vi "Move.vi"(8 "error in (no error)":errorcluster, 11 "Snake in":refnum<class "Snake.lvclass">) -> (0 "error out":errorcluster, 3 "Snake out":refnum<class "Snake.lvclass">)   [LabVIEW 2019, in "RT_Game.lvlib" / "Snake.lvclass"]
uses:
  Snake.lvclass
  Snake.lvclass/Snake.ctl
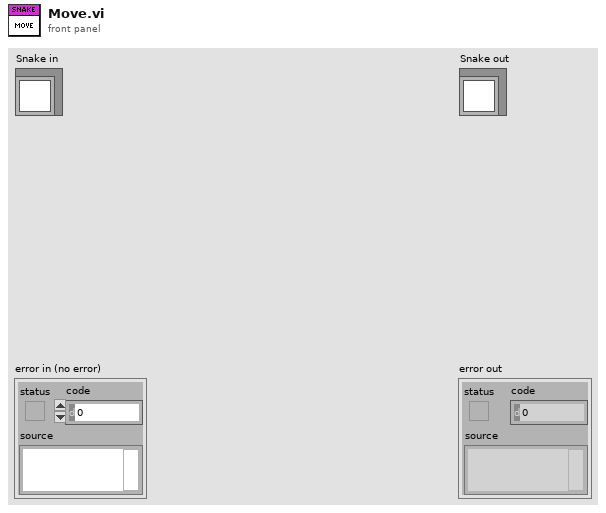
[diagram p1: front panel]
types:
  T1 = typedef "RT_Game.lvlib/Game.lvclass/Coordinate.ctl" = cluster{"x":i16, "y":i16}
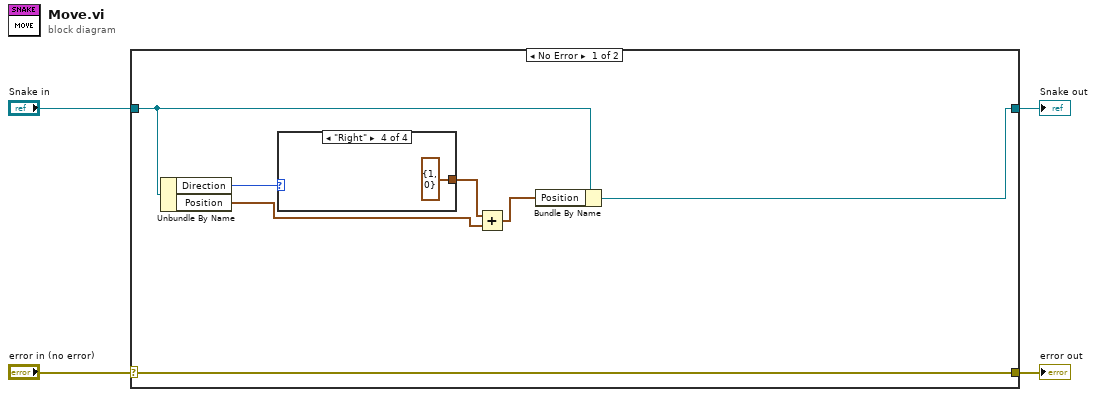
[diagram p0: block diagram]
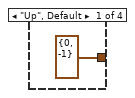
[diagram p2: hidden frame]
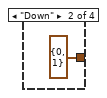
[diagram p3: hidden frame]
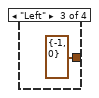
[diagram p4: hidden frame]
diagram:
  n1 = case shown="No Error" "error in (no error)" {
    selector: "error in (no error)" -> [w11 w17]
    tunnel: [w11 w17] -> w3
    tunnel: [w8 w16] -> w1
    tunnel: "Snake in" -> [w10 w16]
    frame No Error {
      n2 = Unbundle By Name(w10) -> ("Direction"=w9:enum16{"Up", "Down", "Left", "Right"}, "Position"=w7:T1)
      n3 = case shown="\"Right\"" w9 {
        tunnel: [cluster{"x":i8, "y":i8} {"x"=0, "y"=-1} ("x") cluster{"x":i8, "y":i8} {"x"=0, "y"=1} ("x") cluster{"x":i8, "y":i8} {"x"=-1, "y"=0} ("x") cluster{"x":i8, "y":i8} {"x"=1, "y"=0} ("x")] -> w6
        frame "Up", Default {
        }
        frame "Down" {
        }
        frame "Left" {
        }
        frame "Right" {
        }
      }
      n4 = Add(x=w6, y=w7) -> (x+y=w5:T1)
      n5 = Bundle By Name(cluster=w10, "Position"=w5) -> (w8:refnum<class "Snake.lvclass">)
    }
    frame Error {
    }
  }
  "error out" <- w3
  "Snake out" <- w1
